vi "FunctDataMgr.Update Data Control Values.vi"(8 "error in (no error)":errorcluster, 11 "FunctDataMgr in":refnum<class "FunctDataMgr.lvclass">) -> (0 "error out":errorcluster, 3 "FunctDataMgr out":refnum<class "FunctDataMgr.lvclass">)   [LabVIEW 2018, in "FunctDataMgr.lvclass"]
uses:
  FunctDataMgr.lvclass
  FunctDataMgr.lvclass/FunctDataMgr.ctl
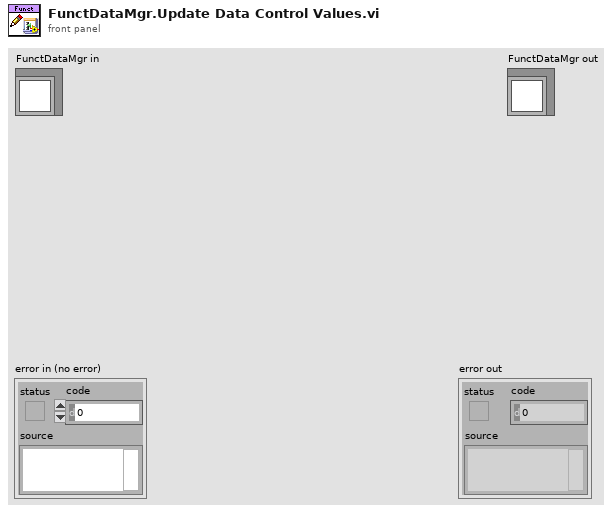
[diagram p1: front panel]
types:
  T1 = typedef "Result.Measurement Item.ctl" = cluster{"Cnt":i32, "Step":string, "Category":string, "Name":string, "Value":string, "Units":string, "LimType":string, "LL":string, "UL":string, "Status":T2, "Code":i32, "Desc":string, "Time":timestamp}
  T2 = typedef "Result.Measurement and Attribute Item Status.ctl" = i32
  T3 = typedef "TestResult.SW Item.ctl" = cluster{"Name":string, "PN":string, "Version":string, "Note":string}
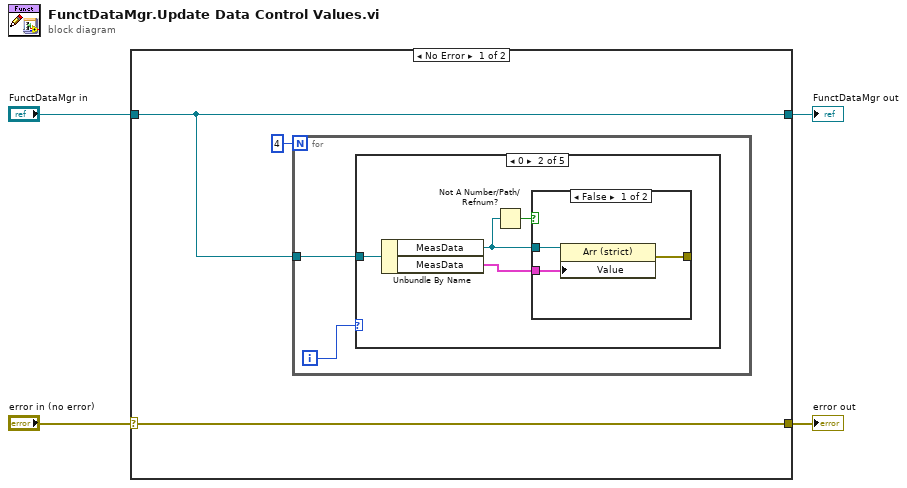
[diagram p0: block diagram]
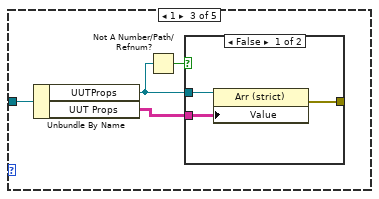
[diagram p4: hidden frame]
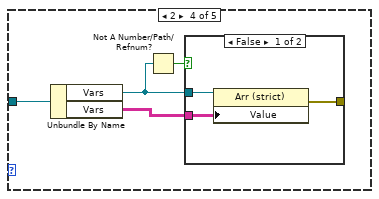
[diagram p6: hidden frame]
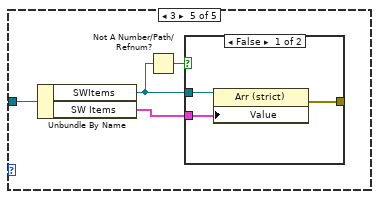
[diagram p8: hidden frame]
diagram:
  n1 = case shown="No Error" "error in (no error)" {
    selector: "error in (no error)" -> [w7 w39]
    tunnel: [w7 w39] -> w3
    tunnel: [w6 w38] -> w1
    tunnel: "FunctDataMgr in" -> [w6 w38]
    frame No Error {
      n2 = for {
        N: 4 -> [_]
        tunnel: w6 -> [w9]
        i -> [w8]
        n3 = case shown="0" w8 {
          tunnel: w9 -> [_ w13 w20 w27 w34]
          frame Default {
          }
          frame 0 {
            n4 = Unbundle By Name(w13) -> ("MeasData"=w12:refnum<vi>, "MeasData"=w11:T1[])
            n5 = Not A Number/Path/Refnum?(number/path/refnum=w12) -> (NaN/Path/Refnum?=w10:bool)
            n6 = case shown="False" w10 {
              tunnel: w12 -> [w16 _]
              tunnel: w11 -> [w15 _]
              tunnel: [w14 _] -> _
              frame False {
                n7 = property class="Arr (strict)"(reference=w16, "Value"=w15) -> (error out=w14:errorcluster)  [unwired: 1 in, 1 out]
              }
              frame True {
              }
            }
          }
          frame 1 {
            n8 = Unbundle By Name(w20) -> ("UUTProps"=w19:refnum<vi>, "UUT Props"=w18:string[][])
            n9 = Not A Number/Path/Refnum?(number/path/refnum=w19) -> (NaN/Path/Refnum?=w17:bool)
            n10 = case shown="False" w17 {
              tunnel: w19 -> [w23 _]
              tunnel: w18 -> [w22 _]
              tunnel: [w21 _] -> _
              frame False {
                n11 = property class="Arr (strict)"(reference=w23, "Value"=w22) -> (error out=w21:errorcluster)  [unwired: 1 in, 1 out]
              }
              frame True {
              }
            }
          }
          frame 2 {
            n12 = Unbundle By Name(w27) -> ("Vars"=w26:refnum<vi>, "Vars"=w25:string[][])
            n13 = Not A Number/Path/Refnum?(number/path/refnum=w26) -> (NaN/Path/Refnum?=w24:bool)
            n14 = case shown="False" w24 {
              tunnel: w26 -> [w30 _]
              tunnel: w25 -> [w29 _]
              tunnel: [w28 _] -> _
              frame False {
                n15 = property class="Arr (strict)"(reference=w30, "Value"=w29) -> (error out=w28:errorcluster)  [unwired: 1 in, 1 out]
              }
              frame True {
              }
            }
          }
          frame 3 {
            n16 = Unbundle By Name(w34) -> ("SWItems"=w33:refnum<vi>, "SW Items"=w32:T3[])
            n17 = Not A Number/Path/Refnum?(number/path/refnum=w33) -> (NaN/Path/Refnum?=w31:bool)
            n18 = case shown="False" w31 {
              tunnel: w33 -> [w37 _]
              tunnel: w32 -> [w36 _]
              tunnel: [w35 _] -> _
              frame False {
                n19 = property class="Arr (strict)"(reference=w37, "Value"=w36) -> (error out=w35:errorcluster)  [unwired: 1 in, 1 out]
              }
              frame True {
              }
            }
          }
        }
      }
    }
    frame Error {
    }
  }
  "error out" <- w3
  "FunctDataMgr out" <- w1
